vi "Obtain Request Events.vi"(8 "error in":errorcluster, 10 "Create New? (F)":bool) -> (0 "error out":errorcluster, 2 "Logger Request Events":T1)   [LabVIEW 2025, in "Logger.lvlib"]
doc: "This VI Obtains/Creates the Requests events that will be used for other modules to communicate with the module that owns this VI. These Requests events will be accessed only via Public API methods for this module.\n\n<b>NOTE</b>: The contents of this VI are automatically generated and modified by the <b>Tools > DQMH Consortium > DQMH</b> utilities. Consider using those utilities instead of making your own modifications to this VI.\n_____\nBased on DQMH Project Template 4.0.0.47.\n_____\nBased on DQMH Dev Tools: Project Template 7.1.0.1503."
uses:
  Logger.lvlib
  Request Events--cluster.ctl
  Stop Argument--cluster.ctl
  Show Panel Argument--cluster.ctl
  Hide Panel Argument--cluster.ctl
  Get Module Execution Status Argument--cluster.ctl
  Show Diagram Argument--cluster.ctl
  Stop Logging Argument--cluster.ctl
  Log Data Argument--cluster.ctl
  Initialize File Argument--cluster.ctl
  Initialize File (Reply Payload)--cluster.ctl
panel:
  # "NOTE: The contents of this VI are automatically generated and modified by the Tools > DQMH Consortium > DQMH utilities. Consider using those utilities instead of making your own modifications to this VI."
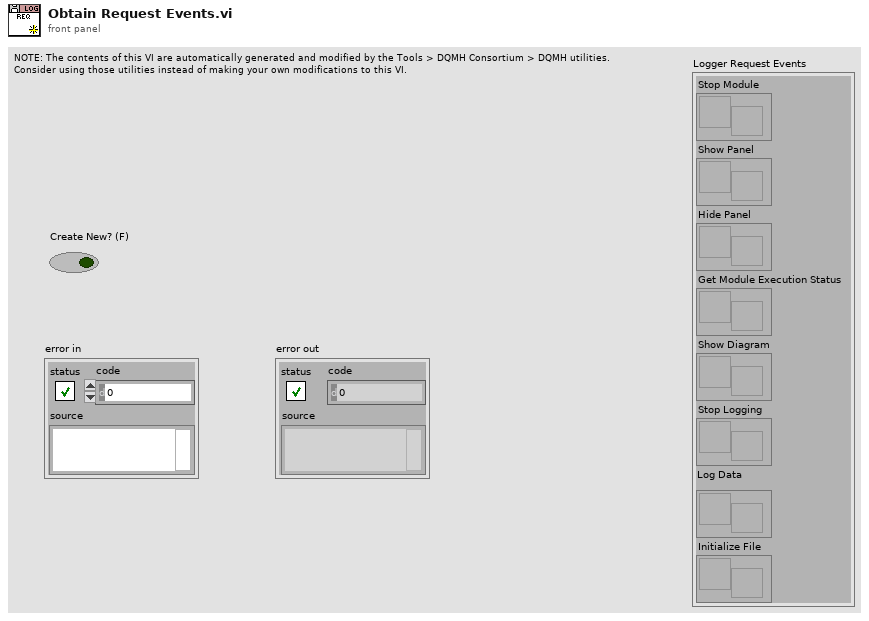
[diagram p1: front panel]
types:
  T1 = typedef "Logger.lvlib/Request Events--cluster.ctl" = cluster{"Stop Module":refnum<user-event>, "Show Panel":refnum<user-event>, "Hide Panel":refnum<user-event>, "Get Module Execution Status":refnum<user-event>, "Show Diagram":refnum<user-event>, "Stop Logging":refnum<user-event>, "Log Data":refnum<user-event>, "Initialize File":refnum<user-event>}
  T2 = typedef "Logger.lvlib/Initialize File Argument--cluster.ctl" = cluster{"Wait Notifier":refnum<notifier>, "wait for reply":bool}
  T3 = typedef "Logger.lvlib/Log Data Argument--cluster.ctl" = cluster{"Waveform":waveform(dbl)}
  T4 = typedef "Logger.lvlib/Stop Logging Argument--cluster.ctl" = cluster{"Boolean":bool}
  T5 = typedef "Logger.lvlib/Hide Panel Argument--cluster.ctl" = cluster{"Hide Panel?":bool}
  T6 = typedef "Logger.lvlib/Show Panel Argument--cluster.ctl" = cluster{"Show Panel?":bool}
  T7 = typedef "Logger.lvlib/Show Diagram Argument--cluster.ctl" = cluster{"Debug?":bool}
  T8 = typedef "Logger.lvlib/Get Module Execution Status Argument--cluster.ctl" = cluster{"Running?":bool}
  T9 = typedef "Logger.lvlib/Stop Argument--cluster.ctl" = cluster{"Origin":string, "Exit via Stop Module Req?":bool, "Wait for Module to stop?":bool}
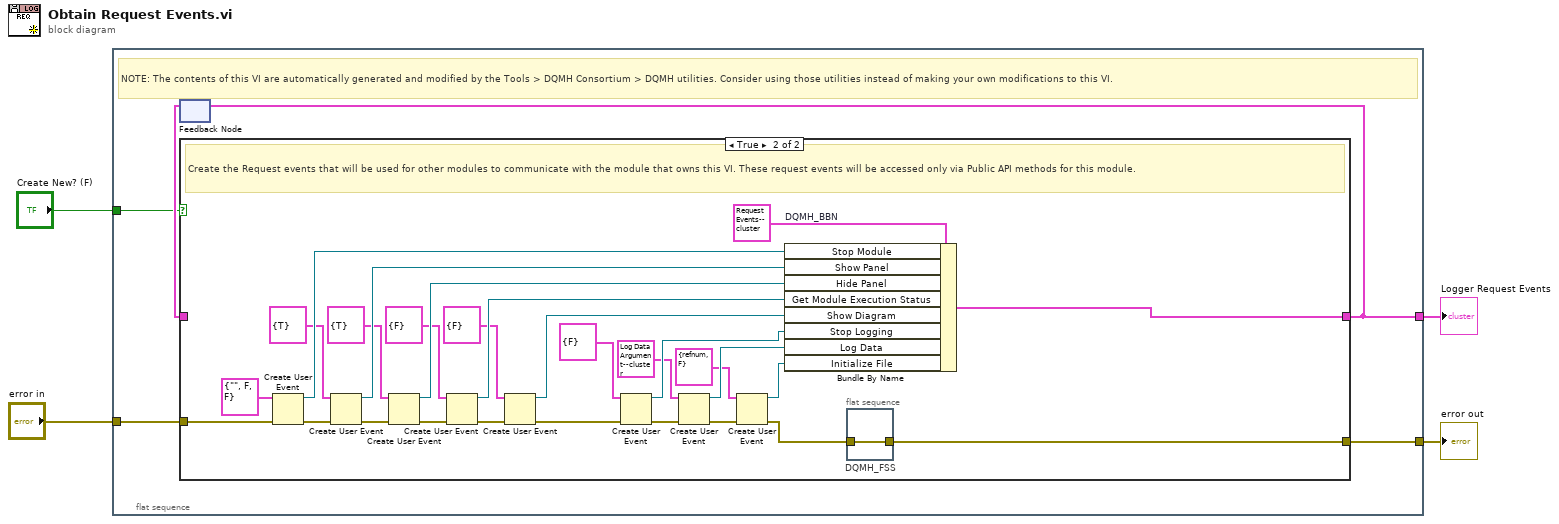
[diagram p0: block diagram]
diagram:
  n1 = flat-sequence {
    tunnel: [w9] -> w4
    tunnel: "error in" -> [w8]
    tunnel: [w6] -> w2
    tunnel: "Create New? (F)" -> [w5]
    frame #0 {
      # "NOTE: The contents of this VI are automatically generated and modified by the Tools > DQMH Consortium > DQMH utilities. Consider using those utilities instead of making your own modifications to this VI."
      n2 = feedback #1() -> (w7:T1)  [unwired: 1 in]
      n3 = case shown="True" w5 {
        tunnel: [w10 w29] -> w9
        tunnel: w8 -> [w10 w39]
        tunnel: [w11 w36] -> w6
        tunnel: w7 -> [w11 _]
        frame False {
          # "Obtain the Request events that were created in a previous call to this VI."
        }
        frame True {
          # "Create the Request events that will be used for other modules to communicate with the module that owns this VI. These request events will be accessed only via Public API methods for this module."
          n4 = Create User Event(user event datatype=T9 {"Origin"="", "Exit via Stop Module Req?"=FALSE, "Wait for Module to stop?"=FALSE} ("Stop Argument"), error in=w39) -> (user event=w37:refnum<user-event>, error out=w34:errorcluster)
          n5 = Create User Event(user event datatype=T6 {"Show Panel?"=TRUE} ("Show Panel Argument"), error in=w34) -> (user event=w33:refnum<user-event>, error out=w32:errorcluster)
          n6 = Create User Event(user event datatype=T5 {"Hide Panel?"=TRUE} ("Hide Panel Argument"), error in=w32) -> (user event=w31:refnum<user-event>, error out=w30:errorcluster)
          n7 = Create User Event(user event datatype=T8 {"Running?"=FALSE} ("Get Module Execution Status Argument"), error in=w30) -> (user event=w27:refnum<user-event>, error out=w28:errorcluster)
          n8 = Create User Event(user event datatype=T7 {"Debug?"=FALSE} ("Show Diagram Argument"), error in=w28) -> (user event=w24:refnum<user-event>, error out=w25:errorcluster)
          n9 = Create User Event(user event datatype=T4 {"Boolean"=FALSE} ("Stop Logging Argument"), error in=w25) -> (user event=w19:refnum<user-event>, error out=w20:errorcluster)
          n10 = Create User Event(user event datatype=T3 {"Waveform"={"t0"=timestamp(0 s since 1904-01-01), "dt"=1.0, "Y"=[]}} ("Log Data to File Argument"), error in=w20) -> (user event=w16:refnum<user-event>, error out=w17:errorcluster)
          n11 = Create User Event(user event datatype=T2 {"Wait Notifier"=refnum, "wait for reply"=FALSE} ("Initialize File Argument"), error in=w17) -> (user event=w13:refnum<user-event>, error out=w14:errorcluster)
          n12 = Bundle By Name "DQMH_BBN"(cluster=T1 {"Stop Module"=refnum, "Show Panel"=refnum, "Hide Panel"=refnum, "Get Module Execution Status"=refnum, "Show Diagram"=refnum, "Stop Logging"=refnum, "Log Data"=refnum, "Initialize File"=refnum} ("output cluster"), "Stop Module"=w37, "Show Panel"=w33, "Hide Panel"=w31, "Get Module Execution Status"=w27, "Show Diagram"=w24, "Stop Logging"=w19, "Log Data"=w16, "Initialize File"=w13) -> (w36:T1)
          n13 = flat-sequence "DQMH_FSS" {
            tunnel: w14 -> [w40]
            tunnel: [w40] -> w29
            frame #0 {
            }
          }
        }
      }
      n14 = feedback-in #1(w6) -> ()
    }
  }
  "Logger Request Events" <- w2
  "error out" <- w4
